vi "Password Input VI with Key Navigation LV2012 NI Verified.vi"(7 "The Password":string="password", 8 "error in (no error)":errorcluster) -> (0 "error out":errorcluster, 1 "Number of Incorrect Responses":i32, 2 "Password Correct?":bool)   [LabVIEW 2018]
doc: "This VI has a password input UI that will allow you to compare the input to a known input value. It is event based so it will trigger off of the enter button on the front panel or either of the two standard Enter keys on the Keyboard.\n\nFor Comments or Improvments go to the Community Post for this Example\nhttp://decibel.ni.com/content/docs/DOC-7222"
panel:
  out "Status":string
  in  "exit":bool
  in  "Enter":bool
  in  "Password Input":string
  # "Overview: This VI has a password input UI that will allow you to compare the input to a known input value.\n\nRequirements: LabVIEW 2012 (or compatible). Hardware: none.\n\nInstructions:\n1. Run the VI.\n2. Try different passwords.\n3. Click Enter after each attempt.\n4. Try password.\n5. Voila."
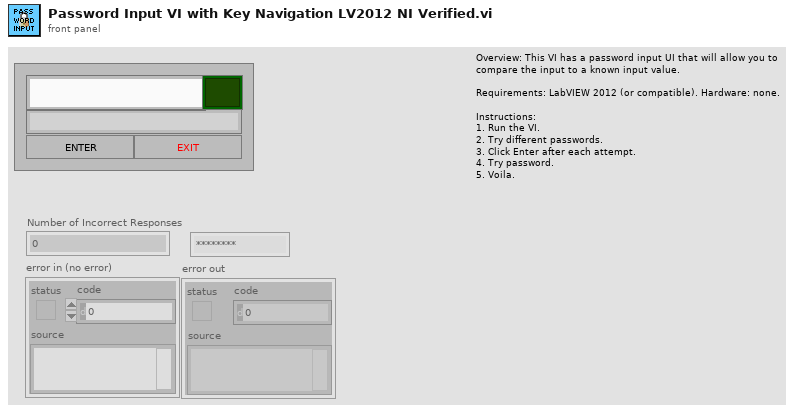
[diagram p1: front panel]
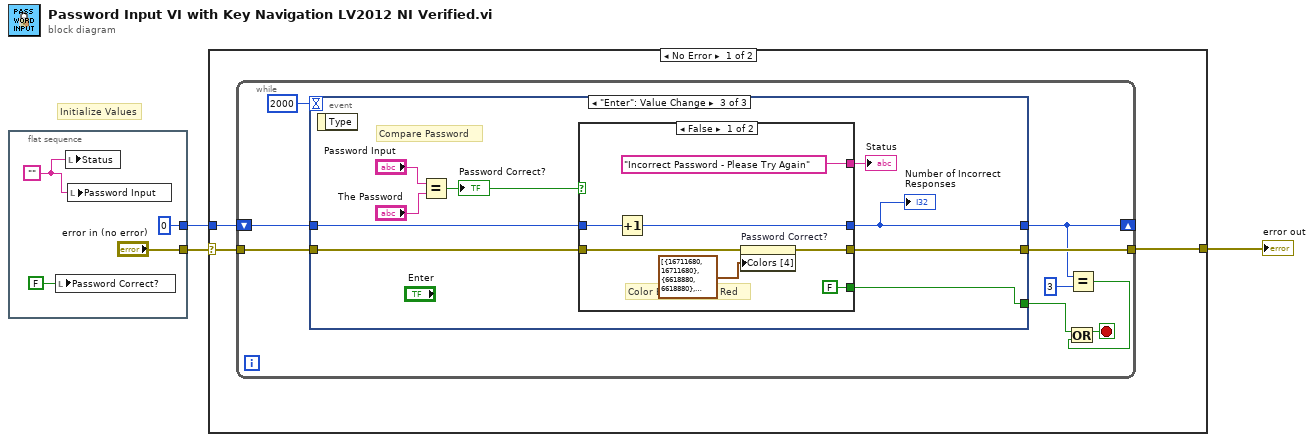
[diagram p0: block diagram]
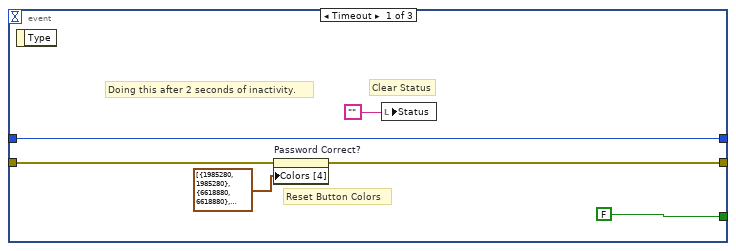
[diagram p2: hidden frame]
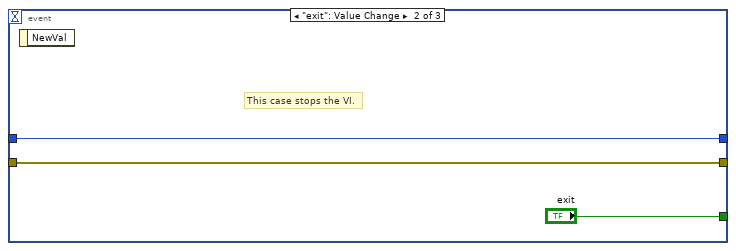
[diagram p3: hidden frame]
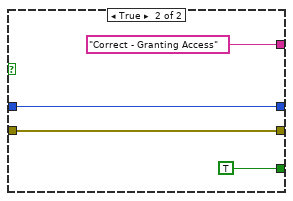
[diagram p4: hidden frame]
diagram:
  # "Initialize Values"
  n1 = flat-sequence {
    tunnel: ["error in (no error)"] -> w2
    tunnel: [0] -> w1
    frame #0 {
      w4 = "" ("Status")
      n2 = local write "Password Correct?"(FALSE ("Passwrod Correct? 2")) -> ()
      n3 = local write "Status"(w4) -> ()
      n4 = local write "Password Input"(w4) -> ()
    }
  }
  n5 = case shown="No Error" w2 {
    selector: w2 -> [w9 w49]
    tunnel: [w10 w49] -> w3
    tunnel: w1 -> [w8 _]
    frame No Error {
      n6 = while {
        shift-right: [w14] -> _
        shift-left: w8 -> [w19]
        tunnel: w9 -> [w17]
        tunnel: [w16] -> w10
        stop <- w13 stop-if-true
        n7 = event shown="[2] \"Enter\": Value Change" {
          selector: _ -> [_ _ _]
          dyn-events: _ -> [_ _ _]
          timeout: 2000 -> [_ _ _]
          tunnel: [FALSE ("exit") "exit" w29] -> w15
          tunnel: w19 -> [w24 w27 w35]
          tunnel: [w24 w27 w33] -> w14
          tunnel: w17 -> [w22 w26 w32]
          tunnel: [w21 w26 w31] -> w16
          event Timeout {
            # "Doing this after 2 seconds of inactivity."
            # "Reset Button Colors"
            # "Clear Status"
            n8 = event-data() -> ()  [unwired: 1 in, 1 out]
            n9 = property on="Password Correct?" class="Bool (strict)"(error in=w22, "Colors [4]"=cluster{u32, u32}[] [{1985280, 1985280}, {6618880, 6618880}, {1985280, 1985280}, {6618880, 6618880}]) -> (error out=w21:errorcluster)  [unwired: 1 in, 1 out]
            n10 = local write "Status"("") -> ()
          }
          event "exit": Value Change {
            # "This case stops the VI."
            n11 = event-data() -> ()  [unwired: 1 in, 1 out]
          }
          event "Enter": Value Change {
            # "Compare Password"
            n12 = event-data() -> ()  [unwired: 1 in, 1 out]
            n13 = Equal?(x="Password Input", y="The Password") -> (x = y?=w34:bool)
            "Password Correct?" <- w34
            n14 = case shown="False" w34 {
              tunnel: ["Incorrect Password - Please Try Again" ("y") "Correct - Granting Access" ("y")] -> w36
              tunnel: w35 -> [w43 w47]
              tunnel: [w42 w47] -> w33
              tunnel: w32 -> [w40 w46]
              tunnel: [w39 w46] -> w31
              tunnel: [FALSE ("exit") TRUE ("exit")] -> w29
              frame False {
                # "Color Enter Button Red"
                n15 = Increment(x=w43) -> (x+1=w42:i32)
                n16 = property on="Password Correct?" class="Bool (strict)"(error in=w40, "Colors [4]"=cluster{u32, u32}[] [{16711680, 16711680}, {6618880, 6618880}, {1985280, 1985280}, {6618880, 6618880}]) -> (error out=w39:errorcluster)  [unwired: 1 in, 1 out]
              }
              frame True {
              }
            }
            "Status" <- w36
            "Number of Incorrect Responses" <- w33
          }
        }
        n17 = Equal?(x=w14, y=3) -> (x = y?=w12:bool)
        n18 = Or(x=w15, y=w12) -> (x .or. y?=w13:bool)
      }
    }
    frame Error {
      # "Do nothing on error."
    }
  }
  "error out" <- w3
